vi "BFSIterator_Init.vi"(0 "object in":refnum<class "BFSIterator.lvclass">, 5 "Error In":errorcluster) -> (14 "object out":refnum<class "BFSIterator.lvclass">, 19 "Error Out":errorcluster)   [LabVIEW 2024, in "BFSIterator.lvclass"]
uses:
  BFSIterator.lvclass
  BFSIterator.lvclass/BFSIterator.ctl
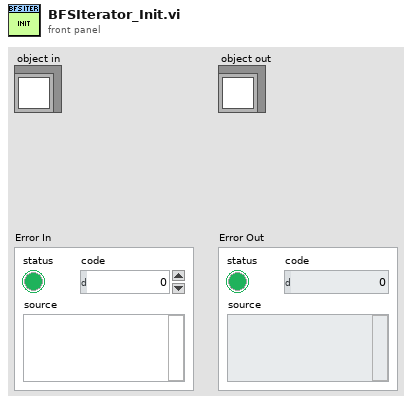
[diagram p1: front panel]
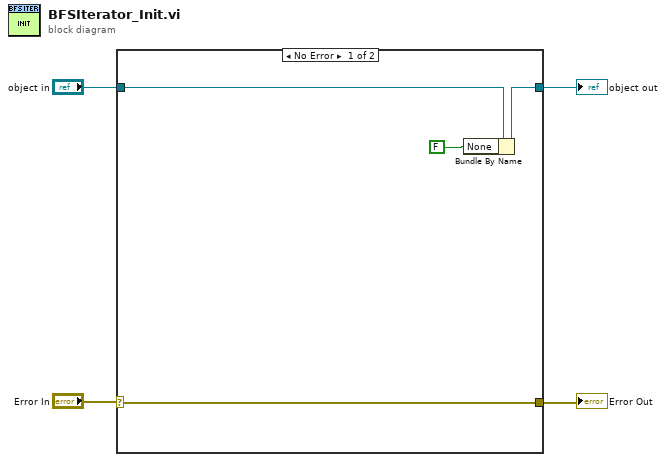
[diagram p0: block diagram]
diagram:
  n1 = case shown="No Error" "Error In" {
    selector: "Error In" -> [w5 w9]
    tunnel: "object in" -> [w8 w10]
    tunnel: [w7 w10] -> w3
    tunnel: [w5 w9] -> w1
    frame No Error {
      n2 = Bundle By Name(cluster=w8, "None"=FALSE) -> (w7:refnum<class "BFSIterator.lvclass">)
    }
    frame Error {
    }
  }
  "object out" <- w3
  "Error Out" <- w1
